vi "Find Node.vi"(8 "error in (no error)":errorcluster, 10 "UID":string, 11 "Base Tree in":refnum<class "Base Tree.lvclass">) -> (0 "error out":errorcluster, 1 "Found?":bool, 2 "Node":refnum<class "Generic Node.lvclass">, 3 "Base Tree out":refnum<class "Base Tree.lvclass">)   [LabVIEW 2017, in "opcua.lvlib" / "Browser Core.lvlib" / "Base Tree.lvclass"]
doc: "Find and return node by UID"
uses:
  Base Tree.lvclass
  Node Classes/Generic Node/Generic Node.lvclass
  Base Tree.lvclass/Base Tree.ctl
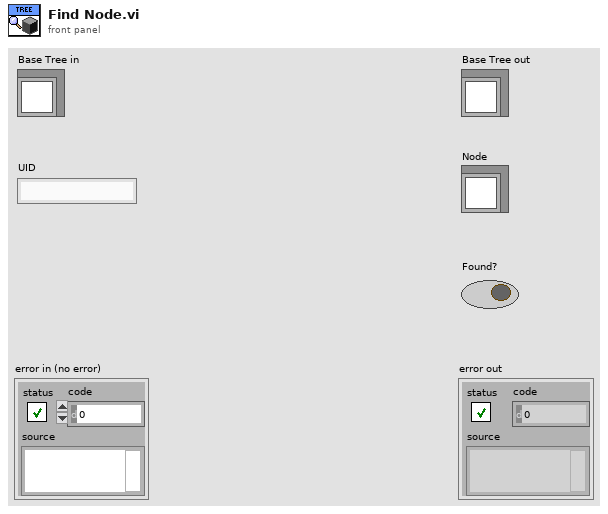
[diagram p1: front panel]
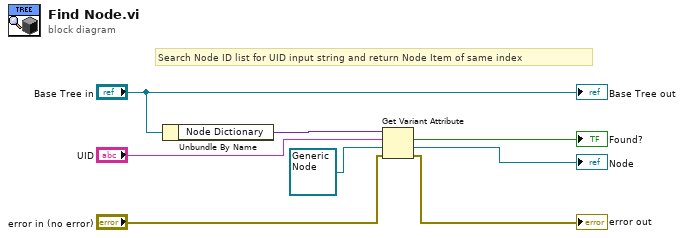
[diagram p0: block diagram]
diagram:
  # "Search Node ID list for UID input string and return Node Item of same index"
  n1 = Unbundle By Name("Base Tree in") -> ("Node Dictionary"=w7:variant)
  n2 = Get Variant Attribute(Variant=w7, name="UID", default value (empty Variant)=refnum<class "Generic Node.lvclass"> refnum ("Node"), error in="error in (no error)") -> (found=→"Found?":bool, value=→"Node":refnum<class "Generic Node.lvclass">, error out=→"error out":errorcluster)  [unwired: 1 out]
  "Base Tree out" <- "Base Tree in"
